vi "WriteDialogStatus.vi"(8 "error in (no error)":errorcluster, 9 "BuildType":T1 items=["simple", "Dialog", "PVUpdate", "Dialog&PV", "Asynch", "AsynchDial"], 10 "Configure Dialog?":bool, 11 "ClassReference":refnum<vi>) -> (0 "error out":errorcluster, 3 "reference out":refnum<vi>)   [LabVIEW 2016, in "CS++Actor.lvlib" / "CS++Actor.lvclass"]
uses:
  CS++Actor.lvclass
  CSPP_MessageMakerMain/BuildType.ctl
  CSPP_MessageMakerMain/CS++MessageMakerMain.lvclass
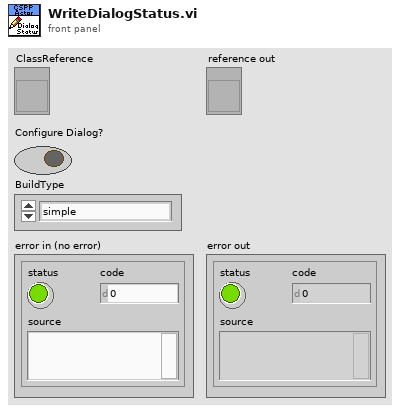
[diagram p1: front panel]
types:
  T1 = typedef "CS++MessageMakerMain.lvlib/CS++MessageMakerMain.lvclass/BuildType.ctl" = u16
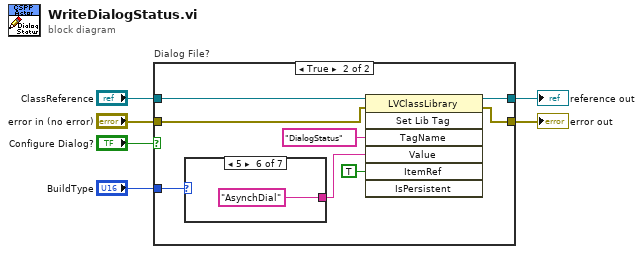
[diagram p0: block diagram]
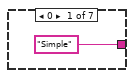
[diagram p3: hidden frame]
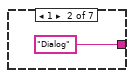
[diagram p4: hidden frame]
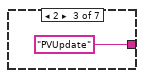
[diagram p5: hidden frame]
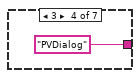
[diagram p6: hidden frame]
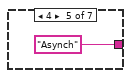
[diagram p7: hidden frame]
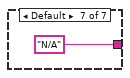
[diagram p8: hidden frame]
diagram:
  n1 = case "Dialog File?" shown="True" "Configure Dialog?" {
    tunnel: "ClassReference" -> [w8 w15]
    tunnel: "error in (no error)" -> [w7 w14]
    tunnel: [w7 w13] -> w3
    tunnel: [w8 w12] -> w2
    tunnel: "BuildType" -> [_ w11]
    frame False {
    }
    frame True {
      n2 = case shown="5" w11 {
        tunnel: ["Simple" ("Tag Name") "Dialog" ("Tag Name") "PVUpdate" ("Tag Name") "PVDialog" ("Tag Name") "Asynch" ("Tag Name") "AsynchDial" ("Tag Name") "N/A" ("Tag Name")] -> w10
        frame 0 {
        }
        frame 1 {
        }
        frame 2 {
        }
        frame 3 {
        }
        frame 4 {
        }
        frame 5 {
        }
        frame Default {
        }
      }
      n3 = invoke class="LVClassLibrary" method="Set Lib Tag"(reference=w15, error in=w14, "TagName"="DialogStatus" ("Tag Name"), "Value"=w10, "ItemRef"=TRUE ("Is Persistent")) -> (reference out=w12:refnum<vi>, error out=w13:errorcluster)  [unwired: 2 in, 5 out]
    }
  }
  "error out" <- w3
  "reference out" <- w2
